vi "Impedance_SingleStats.vi"(4 "Save Every\nRun File?":bool, 6 "Save final stats":bool, 8 "Saving Cluster":T3={"Experiment Title"="Experiment Title", "Save Path"=path "C:/Users/Human-MPI/Desktop/Temp", "File Name String"="TestStats", "Meta-Data Array"=[1.0]}, 9 "samples":i32=10 format="%#.6p", 10 "LCR Params":T4={"Rg_Vmon"=5000.0, "Rg_Imon"=5000.0, "ESL_Cal"=2.5e-07, "ESR_Cal"=0.0, "Cp_Cal"=0.0, "Rp_Cal"=1000000000.0, "UseCorrection"=FALSE, "R_Shunt"=100.0, "RLoad"=1000000000.0, "RLoad_Meas"=1000000000.0} {"RLoad_Meas" format="%#_6p"; "RLoad" format="%#_6p"; "R_Shunt" format="%#_6p"; "Rg_Vmon" format="%#_6p"; "Rg_Imon" format="%#_6p"; "ESL_Cal" format="%#_6p"; "ESR_Cal" format="%#_6p"; "Cp_Cal" format="%#_6p"; "Rp_Cal" format="%#_6p"}, 11 "Test Params Cluster":T5={"Test Freq. (Hz)"=25000.0, "Output Signal Amplitude\nVolts Pk"=0.1, "Sampling Time (s)"=0.1, "Sampling Rate (Hz)"=2000000.0, "Output Channel"="PXI1Slot2/ao1", "Current Channel"="PXI1Slot2/ai1", "Voltage Channel"="PXI1Slot2/ai0", "Trigger Channel"="/PXI1Slot2/ao/StartTrigger", "Number of runs"=10} {"Sampling Rate (Hz)" format="%#_6p"}) -> (0 "Debug Cluster":T1 {"VMon-Ampl" format="%.2p"; "IMon-Ampl" format="%.2p"; "THD-VMon" format="%.2p"; "THD-IMon" format="%.2p"; "detected fundamental frequency" format="%.2p"}, 1 "Histogram Graph Phase":T7(graph)={"X Values"=[95.20701436407293, 95.2415389303248, 95.27606349657665, 95.31058806282851, 95.34511262908038, 95.37963719533224, 95.4141617615841, 95.44868632783596, 95.48321089408782, 95.51773546033968], "Histogram: h(x)"=[1, 0, 0, 2, 1, 1, 2, 1, 1, 1]}, 2 "Histogram Graph Mag":T7(graph)={"X Values"=[0.05657083132191394, 0.05658175212173795, 0.05659267292156196, 0.05660359372138597, 0.05661451452120998, 0.05662543532103399, 0.056636356120858, 0.05664727692068201, 0.05665819772050602, 0.056669118520330033], "Histogram: h(x)"=[1, 0, 1, 0, 1, 0, 4, 1, 1, 1]}, 3 "output cluster":T2 {"Mean |Z|" format="%#_6p"; "standard deviation |Z|" format="%#_6p"; "Mean Phase" format="%#_6p"; "standard deviation Phase" format="%#_6p"; "mean Ls" format="%#_6p"; "Standard dev. Ls" format="%#_6p"; "mean Real(Z)" format="%#_6p"; "Std. dev Real(Z)" format="%#_6p"; "mean Cs" format="%#_6p"; "Std. Dev. Cs" format="%#_6p"; "Mean Rp" format="%#_6p"; "Std. Dev. Rp" format="%#_6p"; "Mean Cp" format="%#_6p"; "Std. Dev. Cp" format="%#_6p"}, 5 "Progress":i32(slide)=90 scale=0.0..100.0, 7 "Current Run Results":T6={"|Z|"=0.05656537092200194, "Phase(Z)"=95.45920483054104, "Re(Z)"=-0.005381459479146001, "Imag(Z)"=0.056308801100875626, "Ls"=3.584729613913086e-07, "Cs"=-0.00011305866221997783, "Rp"=-0.5945675517845621, "Cp"=-0.00011203536283595137} {"|Z|" format="%#_6p"; "Phase(Z)" format="%#_6p"; "Re(Z)" format="%#_6p"; "Imag(Z)" format="%#_6p"; "Ls" format="%#_6p"; "Cs" format="%#_6p"; "Rp" format="%#_6p"; "Cp" format="%#_6p"})   [LabVIEW 2022 SP3]
uses:
  <vilib>/Analysis/NI_AALBase.lvlib
panel:
  out "Array":dbl[][](array[numeric])
  in  "Tab Control":enum32{"Input Params", "Output Plots"}(tab)
  out "Test Number":i32=9
  out "Phase Chart":dbl(graph)=95.45920483054104
  out "Real(Z) Chart":dbl(graph)=-0.005381459479146001
  out "Capacitance Chart":dbl(graph)=-0.00011305866221997783
  out "|Z| over time":dbl(graph)=0.05656537092200194
  out "Inductance Chart":dbl(graph)=3.584729613913086e-07
  # "Will create as many files as there are number of runs\n(Not typical)"
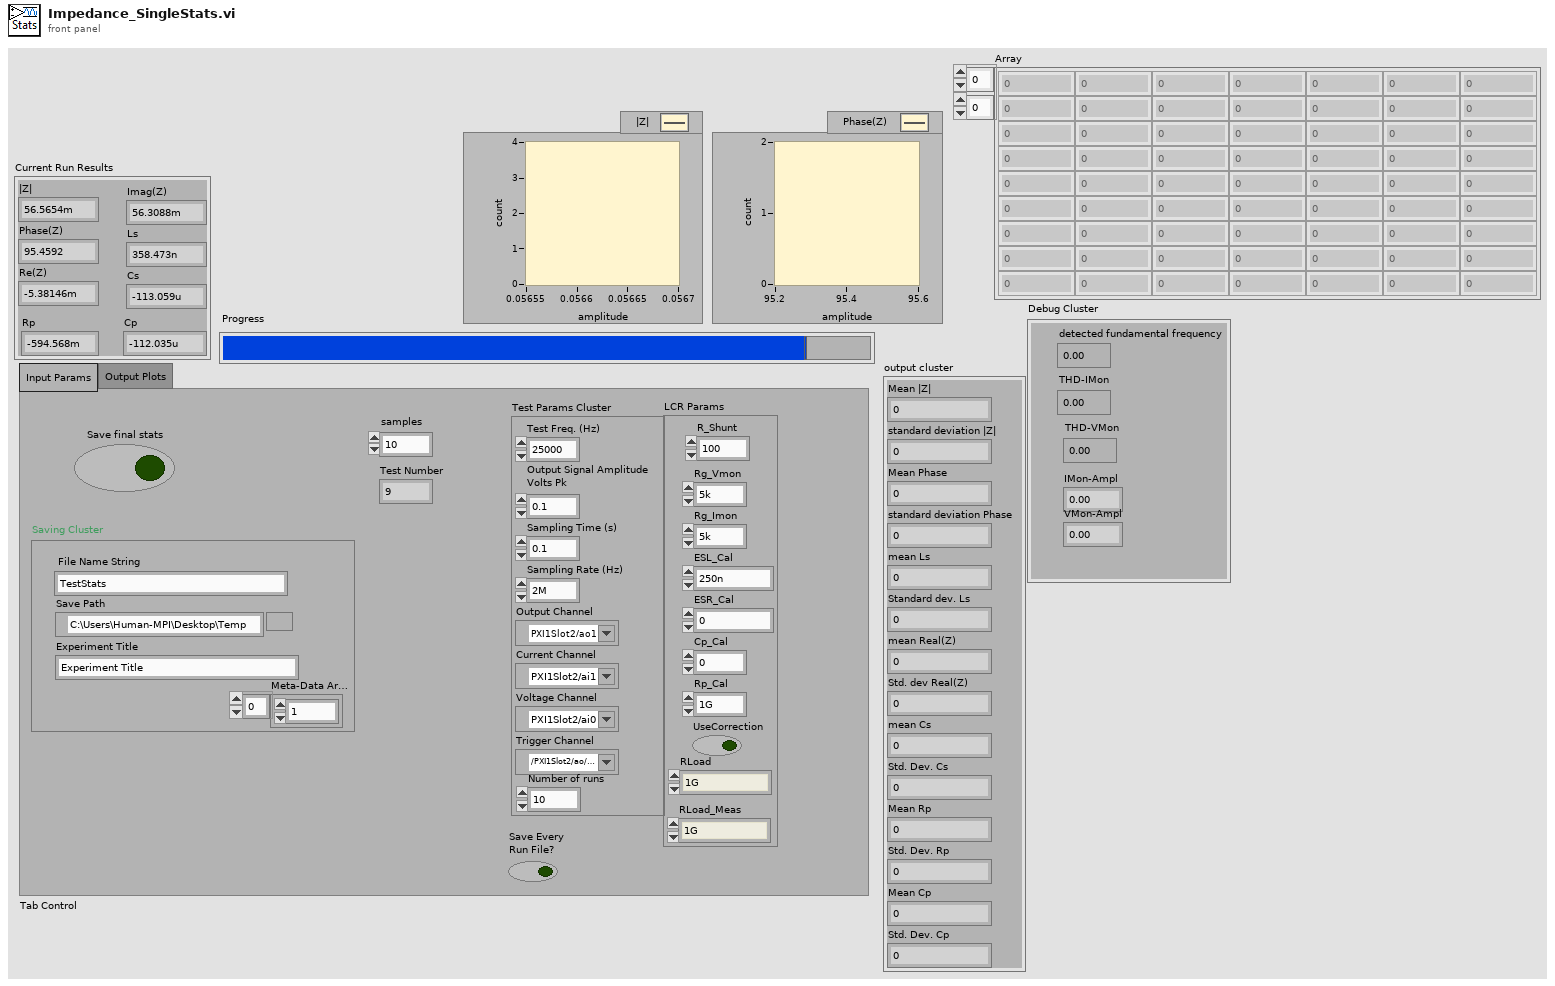
[diagram p1: front panel]
types:
  T1 = cluster{"detected fundamental frequency":dbl, "THD-IMon":dbl, "THD-VMon":dbl, "IMon-Ampl":dbl, "VMon-Ampl":dbl}
  T2 = cluster{"Mean |Z|":dbl, "standard deviation |Z|":dbl, "Mean Phase":dbl, "standard deviation Phase":dbl, "mean Ls":dbl, "Standard dev. Ls":dbl, "mean Real(Z)":dbl, "Std. dev Real(Z)":dbl, "mean Cs":dbl, "Std. Dev. Cs":dbl, "Mean Rp":dbl, "Std. Dev. Rp":dbl, "Mean Cp":dbl, "Std. Dev. Cp":dbl}
  T3 = cluster{"Experiment Title":string, "Save Path":path, "File Name String":string, "Meta-Data Array":dbl[]}
  T4 = cluster{"Rg_Vmon":dbl, "Rg_Imon":dbl, "ESL_Cal":dbl, "ESR_Cal":dbl, "Cp_Cal":dbl, "Rp_Cal":dbl, "UseCorrection":bool, "R_Shunt":dbl, "RLoad":dbl, "RLoad_Meas":dbl}
  T5 = cluster{"Test Freq. (Hz)":dbl, "Output Signal Amplitude\nVolts Pk":dbl, "Sampling Time (s)":dbl, "Sampling Rate (Hz)":dbl, "Output Channel":tag, "Current Channel":tag, "Voltage Channel":tag, "Trigger Channel":tag, "Number of runs":i32}
  T6 = cluster{"|Z|":dbl, "Phase(Z)":dbl, "Re(Z)":dbl, "Imag(Z)":dbl, "Ls":dbl, "Cs":dbl, "Rp":dbl, "Cp":dbl}
  T7 = cluster{"X Values":dbl[], "Histogram: h(x)":i32[]}
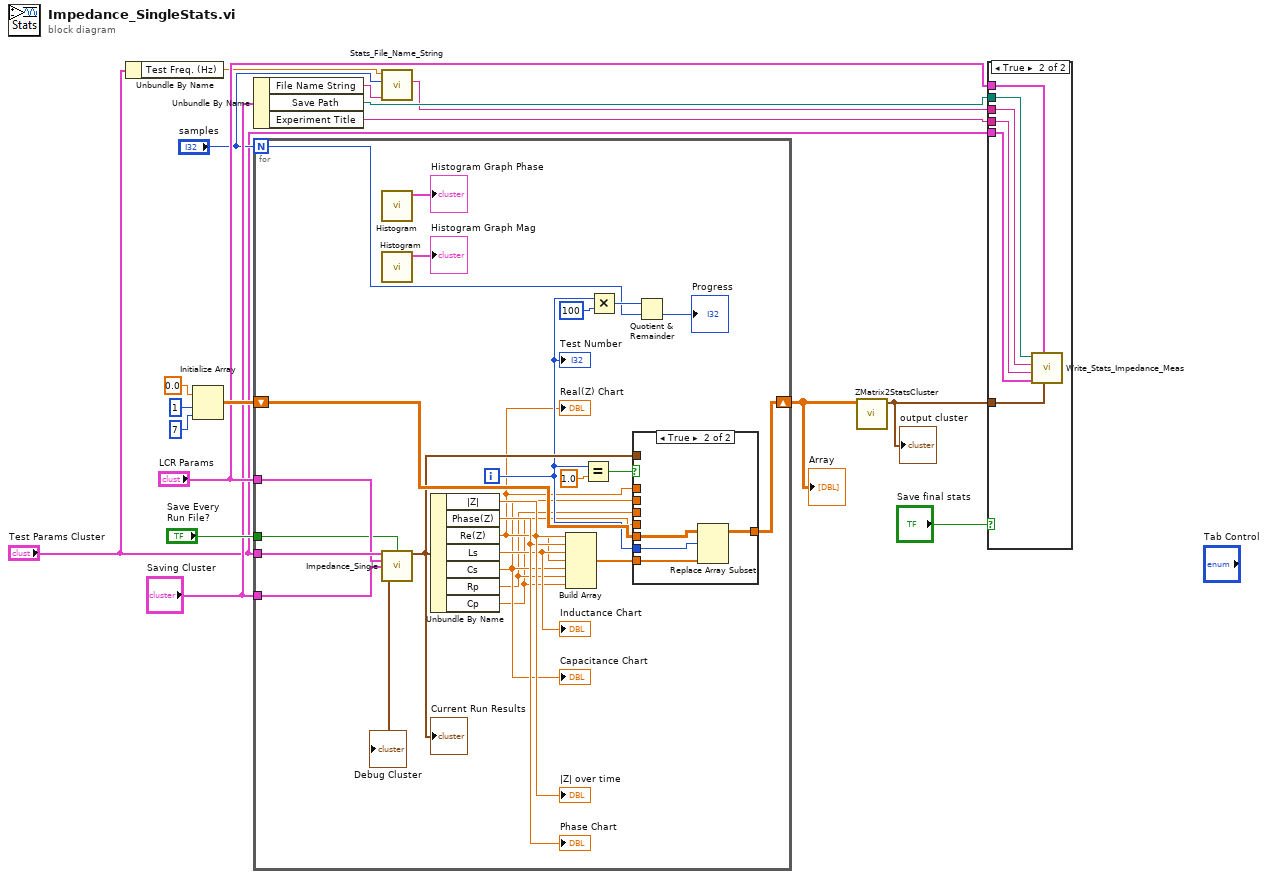
[diagram p0: block diagram]
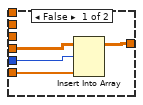
[diagram p2: hidden frame]
diagram:
  n1 = Unbundle By Name("Test Params Cluster") -> ("Test Freq. (Hz)"=w5:dbl)
  n2 = Initialize Array(0.0 ("element"), 1 ("dimension size"), 7 ("dimension size")) -> (w16:dbl[][])
  n3 = Unbundle By Name("Saving Cluster") -> ("File Name String"=w8:string, "Save Path"=w10:path, "Experiment Title"=w11:string)
  n4 = for {
    N: "samples" -> [w29]
    shift-right: [w19] -> w2
    shift-left: w16 -> [w42]
    tunnel: "Test Params Cluster" -> [w37]
    tunnel: "LCR Params" -> [w36]
    tunnel: "Save Every\nRun File?" -> [w35]
    tunnel: "Saving Cluster" -> [w28]
    i -> [w30]
    n5 = call <vilib>:"Histogram.vi"() -> ("Histogram Graph"=→"Histogram Graph Phase":T7)  [unwired: 8 in, 3 out]
    n6 = call <vilib>:"Histogram.vi"() -> ("Histogram Graph"=→"Histogram Graph Mag":T7)  [unwired: 8 in, 3 out]
    n7 = call "Impedance_Single.vi"("Test Params Cluster"=w37, "SaveFile?"=w35, "LCR Params"=w36, "Saving Cluster"=w28) -> ("Mean Signal\nImpedance cluster"=w34:T6, "Debug Cluster"=→"Debug Cluster":T1)  [unwired: 9 in, 1 out]
    "Current Run Results" <- w34
    n8 = Unbundle By Name(w34) -> ("|Z|"=w27:dbl, "Phase(Z)"=w26:dbl, "Re(Z)"=w24:dbl, "Ls"=w25:dbl, "Cs"=w23:dbl, "Rp"=w22:dbl, "Cp"=w21:dbl)
    "|Z| over time" <- w27
    "Real(Z) Chart" <- w24
    "Phase Chart" <- w26
    "Inductance Chart" <- w25
    "Capacitance Chart" <- w23
    n9 = Build Array(w27, w26, w25, w24, w23, w22, w21) -> (w20:dbl[])
    n10 = Equal?(x=w30, y=1.0) -> (x = y?=w39:bool)
    n11 = Multiply(x=w30, y=100) -> (x*y=w31:i32)
    n12 = case shown="True" w39 {
      tunnel: w42 -> [w46 w50]
      tunnel: w30 -> [w44 w48]
      tunnel: [w45 w49] -> w19
      tunnel: w34 -> [_ _]
      tunnel: w23 -> [_ _]
      tunnel: w24 -> [_ _]
      tunnel: w22 -> [_ _]
      tunnel: w21 -> [_ _]
      tunnel: w20 -> [w43 w47]
      frame False {
        n13 = Insert Into Array(array=w46, index (row)=w44, new element=w43) -> (w45:dbl[][])  [unwired: 1 in]
      }
      frame True {
        n14 = Replace Array Subset(array=w50, new element=w47, index (row)=w48) -> (w49:dbl[][])  [unwired: 1 in]
      }
    }
    n15 = Quotient & Remainder(x=w31, y=w29) -> (floor(x/y)=→"Progress":i32)  [unwired: 1 out]
    "Test Number" <- w30
  }
  "Array" <- w2
  n16 = call "Stats_File_Name_String.vi"("String"=w8, "N"="samples", "TestFreq"=w5) -> ("Output string"=w4:string)  [unwired: 8 in]
  n17 = call "ZMatrix2StatsCluster.vi"("Array"=w2) -> ("output cluster 2"=w1:T2)  [unwired: 10 in]
  "output cluster" <- w1
  n18 = case shown="True" "Save final stats" {
    tunnel: "LCR Params" -> [_ w56]
    tunnel: "Test Params Cluster" -> [_ w55]
    tunnel: w11 -> [_ w54]
    tunnel: w4 -> [_ w53]
    tunnel: w10 -> [_ w52]
    tunnel: w1 -> [_ w51]
    frame False {
    }
    frame True {
      n19 = call "Write_Stats_Impedance_Meas.vi"("Output Stats Cluster"=w51, "Compensation and Gain"=w56, "Test Params Cluster"=w55, "Experiment Title"=w54, "File Name String"=w53, "Path"=w52) -> ()  [unwired: 6 in]
    }
  }
